vi "D寄存器输出计算.vi"(11 "字符串":string="\u000234127856\u0003A7") -> (3 "输出":u16[](array[numeric]))   [LabVIEW 2014]
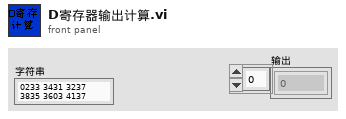
[diagram p1: front panel]
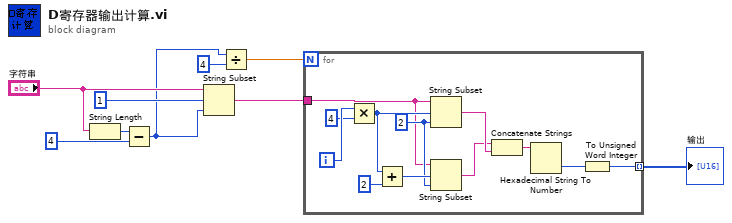
[diagram p0: block diagram]
diagram:
  n1 = String Length(string="字符串") -> (length=w8:i32)
  n2 = Subtract(x=w8, y=4) -> (x-y=w4:i32)
  n3 = String Subset(string="字符串", offset (0)=1 ("偏移量(0)"), length (rest)=w4) -> (substring=w5:string)
  n4 = Divide(x=w4, y=4) -> (x/y=w2:dbl)
  n5 = for {
    N: w2 -> [_]
    tunnel: w5 -> [w15]
    tunnel: [w10] -> w1 mode=indexing
    i -> [w21]
    w16 = 2 ("长度（剩余）")
    n6 = Multiply(x=w21, y=4) -> (x*y=w19:i32)
    n7 = Add(x=w19, y=2 ("长度（剩余）")) -> (x+y=w18:i32)
    n8 = String Subset(string=w15, offset (0)=w19, length (rest)=w16) -> (substring=w14:string)
    n9 = String Subset(string=w15, offset (0)=w18, length (rest)=w16) -> (substring=w13:string)
    n10 = Concatenate Strings(w13, w14) -> (w12:string)
    n11 = Hexadecimal String To Number(string=w12) -> (number=w11:u32)  [unwired: 2 in, 1 out]
    n12 = To Unsigned Word Integer(number=w11) -> (unsigned 16bit integer=w10:u16)
  }
  "输出" <- w1
